vi "RSZVB Get Pulse Train Segment State.vi"(8 "error in (no error)":errorcluster {"code" format="%.0x"}, 9 "Segment (1)":i32=1, 10 "Channel (1)":i32=1, 11 "VISA session":refnum<visa-resource-name>) -> (0 "error out":errorcluster {"code" format="%.0x"}, 1 "Segment State":bool, 3 "dup VISA session":refnum<visa-resource-name>)   [LabVIEW 2011]
doc: "This VI returns the state of the pulse train segment.\n\nNote(s):\n\n(1) This VI is available only with option R&S ZVA-K27.\n\nRemote-control command(s):\n[SENSe<Ch>:]PULSe:GENerator<gen_no>:TRAin:SEGMent<Seg>[:STATe]?"
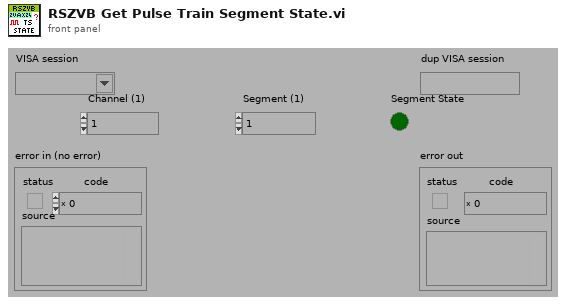
[diagram p1: front panel]
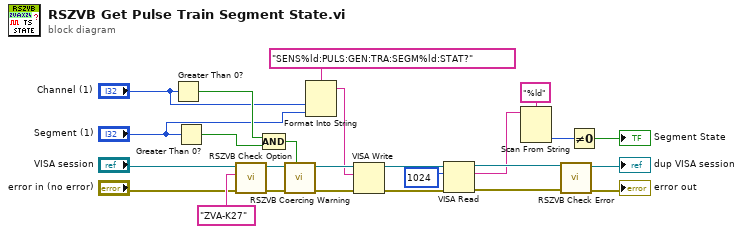
[diagram p0: block diagram]
diagram:
  n1 = Greater Than 0?(x="Channel (1)") -> (x > 0?=w17:bool)
  n2 = Greater Than 0?(x="Segment (1)") -> (x > 0?=w3:bool)
  n3 = call "RSZVB Check Option.vi"("error in (no error)"="error in (no error)", "Options"="ZVA-K27", "VISA session"="VISA session") -> ("error out"=w21:errorcluster, "dup VISA session"=w20:refnum<visa-resource-name>)  [unwired: 7 in]
  n4 = Compound Arithmetic op=AND(w17, w3) -> (w19:bool)
  n5 = call "RSZVB Coercing Warning.vi"("In Range?"=w19, "error in (no error)"=w21, "VISA session"=w20) -> ("error out"=w24:errorcluster, "dup VISA session"=w25:refnum<visa-resource-name>)  [unwired: 7 in]
  n6 = Format Into String(format string="SENS%ld:PULS:GEN:TRA:SEGM%ld:STAT?", "Channel (1)", "Segment (1)") -> (resulting string=w23:string)  [unwired: 2 in, 1 out]
  n7 = VISA Write(VISA resource name=w25, write buffer=w23, error in (no error)=w24) -> (VISA resource name out=w15:refnum<visa-resource-name>, error out=w14:errorcluster)  [unwired: 1 out]
  n8 = VISA Read(VISA resource name=w15, byte count=u32 1024 ("byte count (0)"), error in (no error)=w14) -> (VISA resource name out=w13:refnum<visa-resource-name>, read buffer=w7:string, error out=w12:errorcluster)  [unwired: 1 out]
  n9 = Scan From String(format string="%ld", input string=w7) -> (output 1=w5:i32)  [unwired: 3 in, 3 out]
  n10 = call "RSZVB Check Error.vi"("error in (no error)"=w12, "VISA session"=w13) -> ("error out"=→"error out":errorcluster, "dup VISA session"=→"dup VISA session":refnum<visa-resource-name>)  [unwired: 8 in]
  n11 = Not Equal To 0?(x=w5) -> (x != 0?=→"Segment State":bool)
